vi "main.vi"() -> ()   [LabVIEW 2015]
uses:
  <vilib>/Bitlis-MEN/Parallel Stop/Software/Stop_Command.ctl
  test_chamber/Test Chamber/sub/MKS/Product/MFC/Type Definitions/Modbus Action.ctl
  <vilib>/Utility/file.llb/Write Delimited Spreadsheet (string).vi
  <vilib>/Utility/file.llb/Write Delimited Spreadsheet (DBL).vi
panel:
  in  "?":enum32{"Main", "Notes"}(tab)
  in  "submit_note":bool
  out "pv_6":dbl format="%#_3f"
  in  "sp_6":dbl
  in  "slide_6":dbl(slide) scale=0.0..500.0 scale format="%#_6p"
  out "label_6":string
  out "pv_5":dbl format="%#_3f"
  in  "sp_5":dbl
  in  "slide_5":dbl(slide) scale=0.0..500.0 scale format="%#_6p"
  out "label_5":string
  out "pv_4":dbl format="%#_3f"
  in  "sp_4":dbl
  in  "slide_4":dbl(slide) scale=0.0..500.0 scale format="%#_6p"
  out "label_4":string
  out "pv_3":dbl format="%#_3f"
  in  "sp_3":dbl
  in  "slide_3":dbl(slide) scale=0.0..500.0 scale format="%#_6p"
  out "label_3":string
  out "pv_2":dbl format="%#_3f"
  in  "sp_2":dbl
  in  "slide_2":dbl(slide) scale=0.0..10000.0 scale format="%#_1p"
  out "label_2":string
  out "pv_1":dbl format="%#_3f"
  in  "sp_1":dbl
  in  "slide_1":dbl(slide) scale=0.0..20000.0 scale format="%#_6p"
  out "label_1":string
  in  "mfc_activated 6":bool
  in  "mfc_ip 6":string="192.168.2.6"
  in  "mfc_ip 5":string="192.168.2.5"
  in  "mfc_ip 4":string="192.168.2.4"
  in  "mfc_ip 3":string="192.168.2.3"
  in  "mfc_ip 2":string="192.168.2.2"
  in  "mfc_ip1":string="192.168.2.1"
  in  "mfc_label 6":string="MFC6"
  in  "mfc_label 5":string="MFC5"
  in  "mfc_label 4":string="MFC4"
  in  "mfc_label 3":string="MFC3"
  in  "mfc_label 2":string="MFC 2"
  in  "mfc_label1":string="MFC 1"
  in  "mfc_activated 5":bool
  in  "mfc_activated 4":bool
  in  "mfc_activated 3":bool
  in  "mfc_activated 2":bool
  in  "mfc_activated1":bool
  out "?":errorcluster
  in  "Stop Button":bool
  out "Current State":T1(ring)
  in  "freq":u32=250
  in  "Add a note":string
  in  "File Path Control":path=path "E:/MFC Logger"
  out "Notes":string[][](table)
  # "Things to do:\n\n1) Logging\n2) Note taking\n3) Calibration Page/Worksheet"
  # "Label"
  # "IP Address"
  # "Activated?"
  # "MFC 1"
  # "MFC 2"
  # "MFC 3"
  # "MFC 4"
  # "MFC 5"
  # "MFC 6"
  # "Timestamp"
  # "Message"
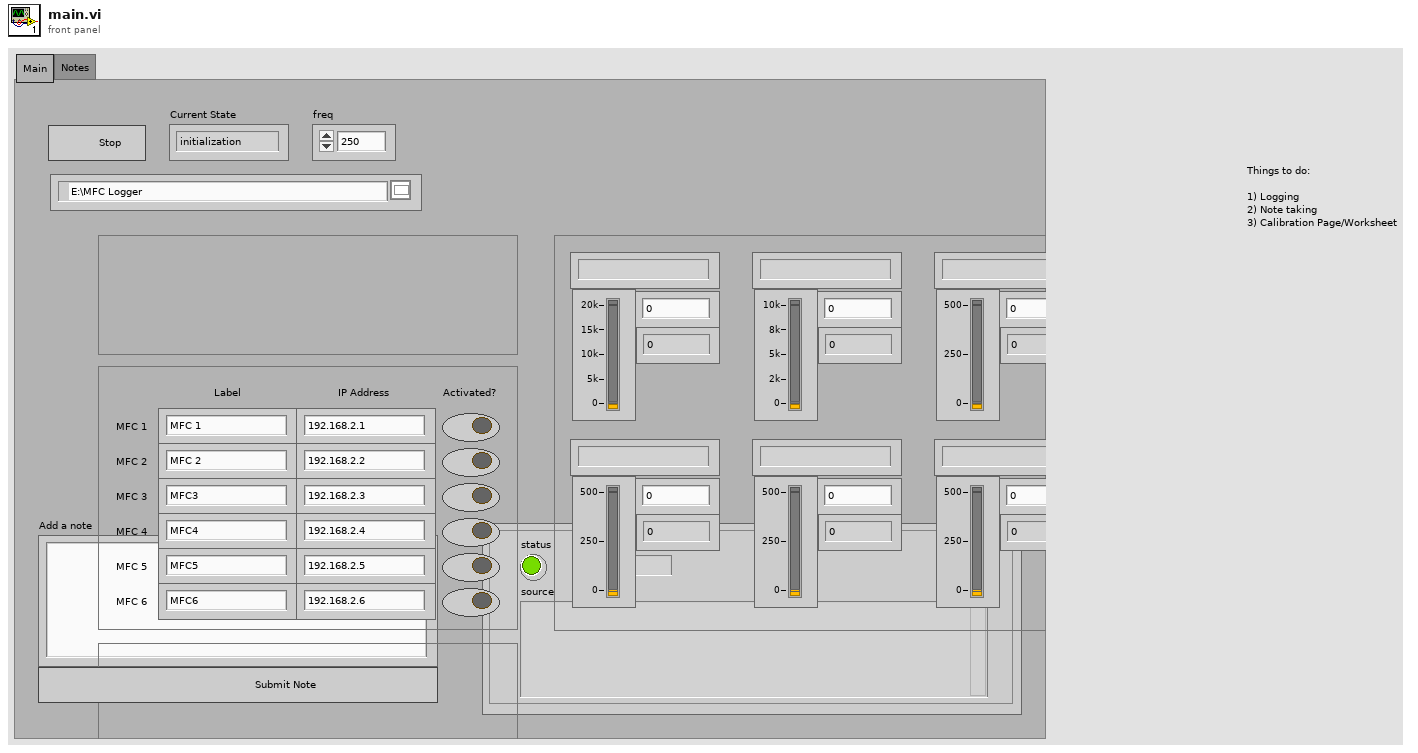
[diagram p1: front panel]
types:
  T1 = enum16{"initialization", "mode_selection", "auto_mode", "manual_mode", "safe_shutdown"}
  T2 = cluster{"Label":string, "IP":string, "Enabled":bool, "TCP Ref":refnum<k5>}[]
  T3 = cluster{"Label":string, "IP":string, "Enabled":bool, "TCP Ref":refnum<k5>}
  T4 = typedef "Stop_Command.ctl" = enum16{"Reset", "Read", "Write", "Close"}
  T5 = typedef "Modbus Action.ctl" = enum16{"Read", "Write"}
  T6 = enum8{"Enabled", "Disabled", "Disabled and Grayed Out"}
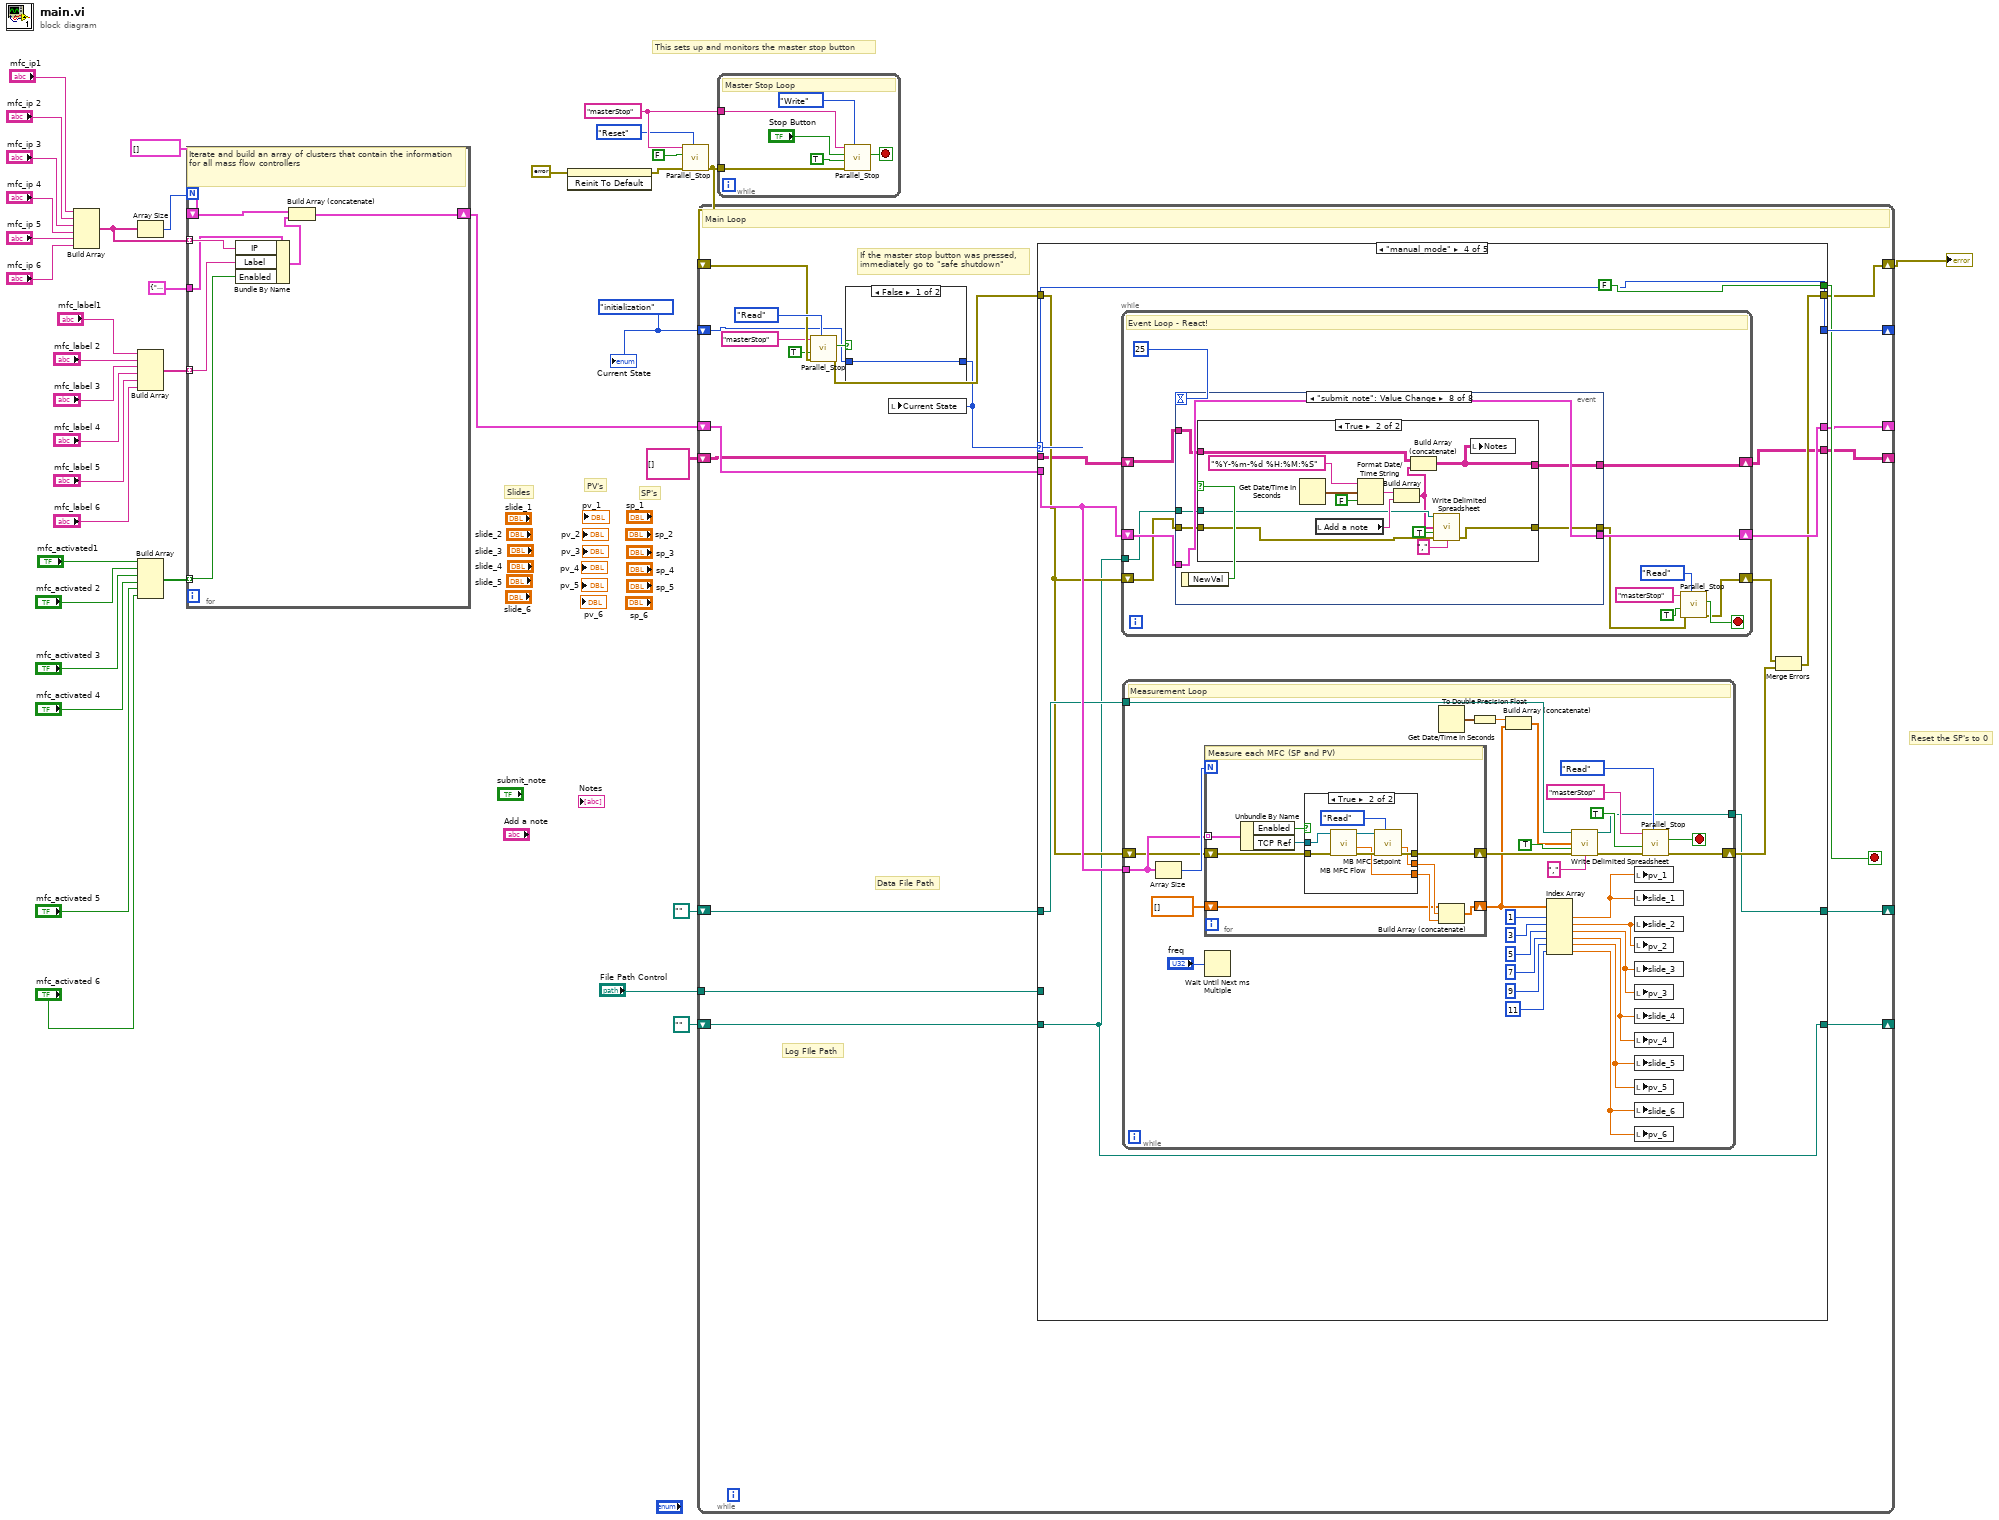
[diagram p0: block diagram]
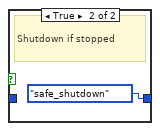
[diagram p2: hidden frame]
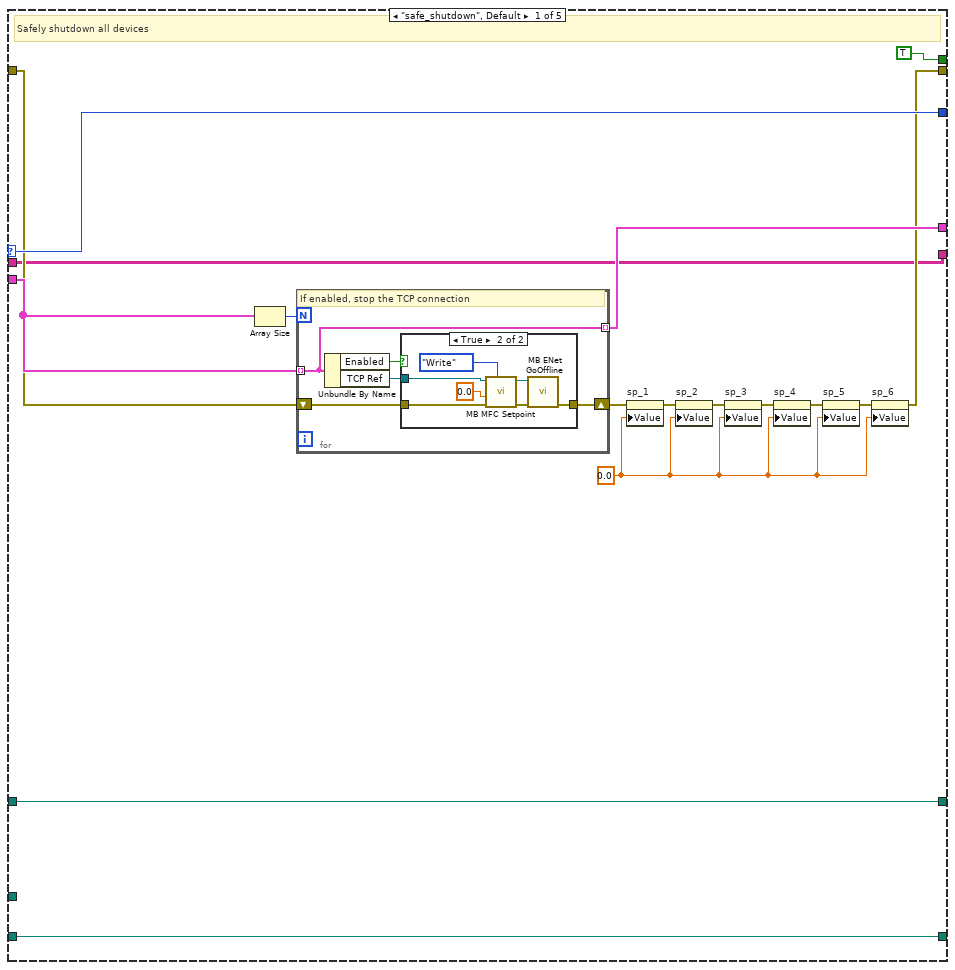
[diagram p3: hidden frame]
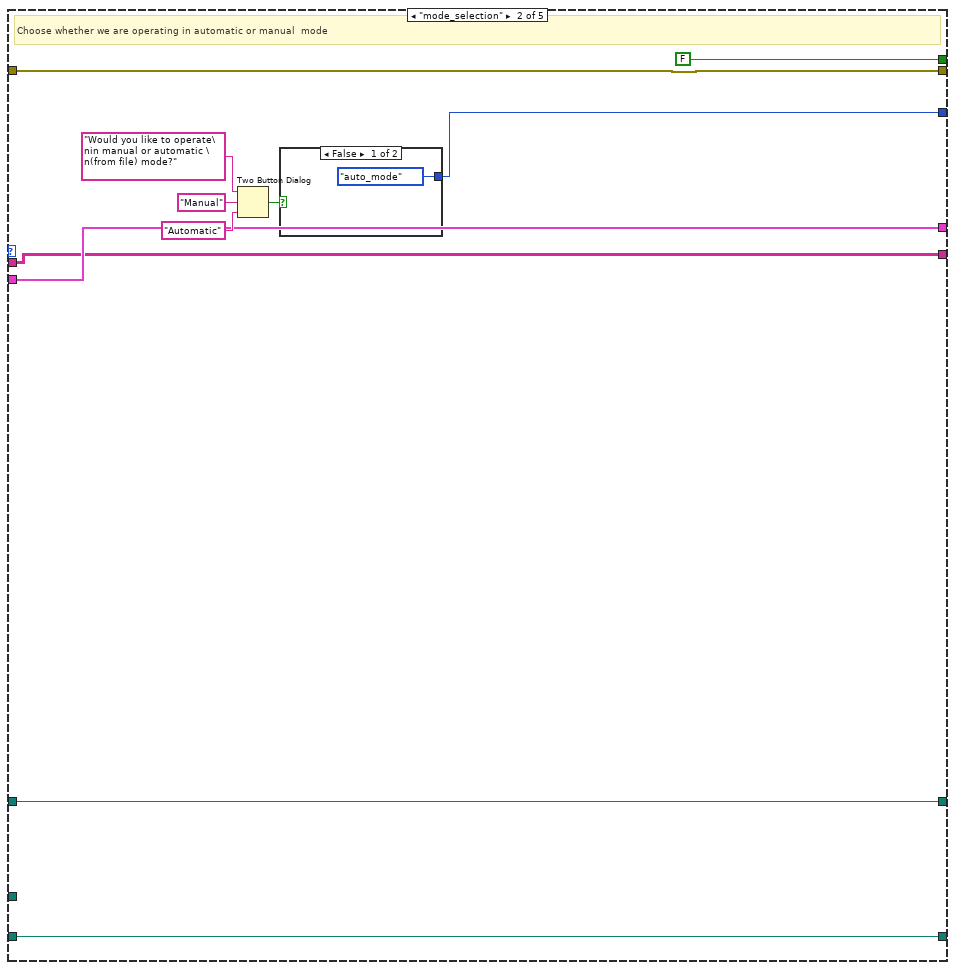
[diagram p5: hidden frame]
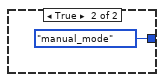
[diagram p6: hidden frame]
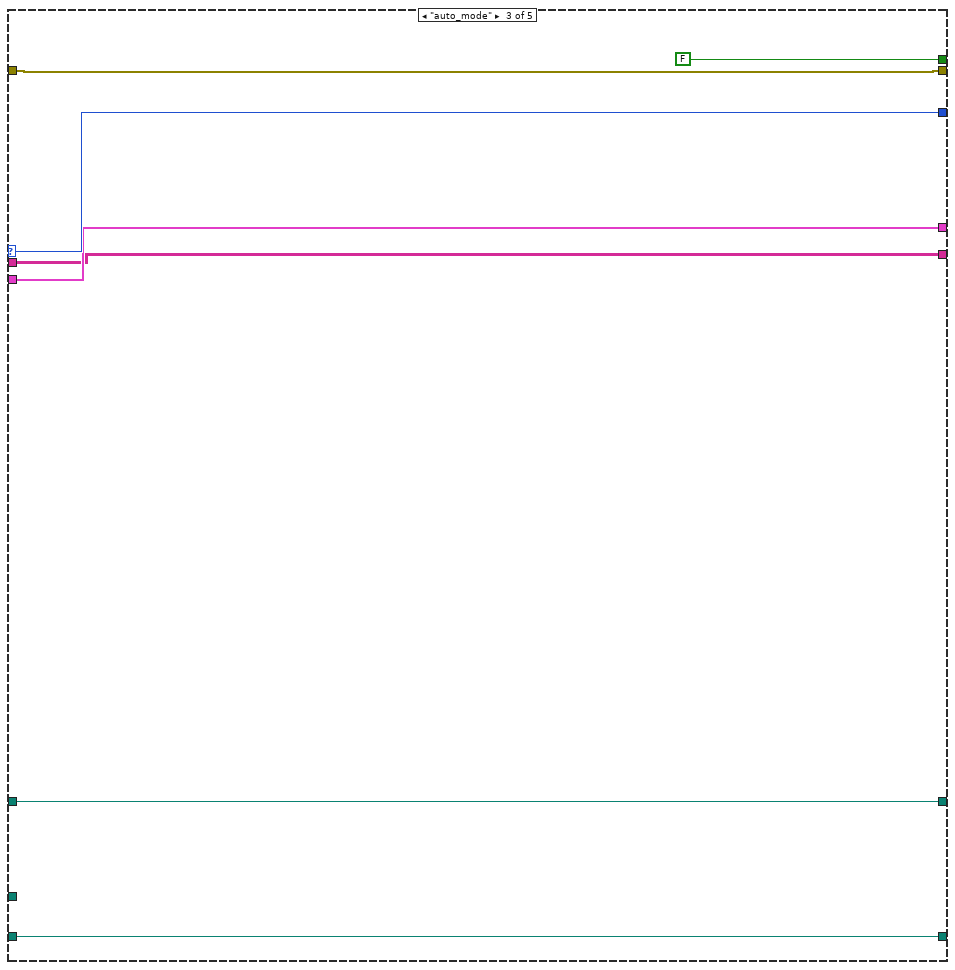
[diagram p7: hidden frame]
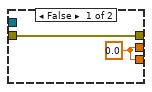
[diagram p8: hidden frame]
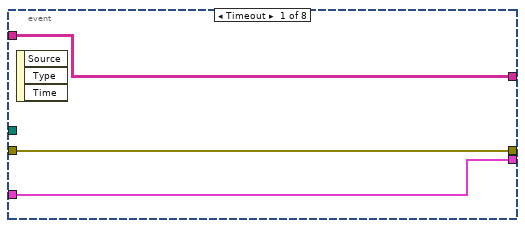
[diagram p9: hidden frame]
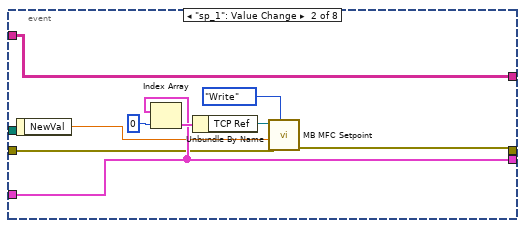
[diagram p10: hidden frame]
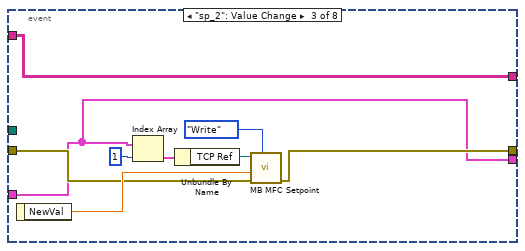
[diagram p11: hidden frame]
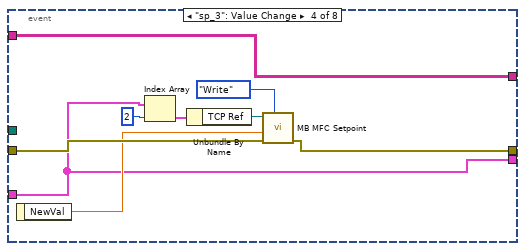
[diagram p12: hidden frame]
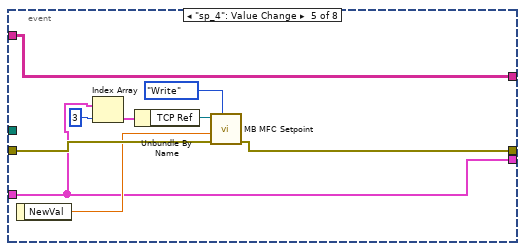
[diagram p13: hidden frame]
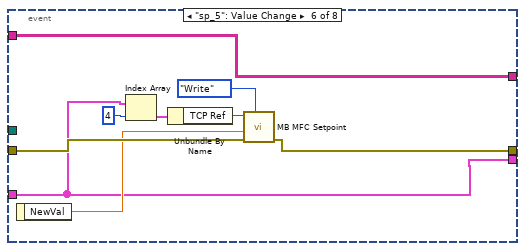
[diagram p14: hidden frame]
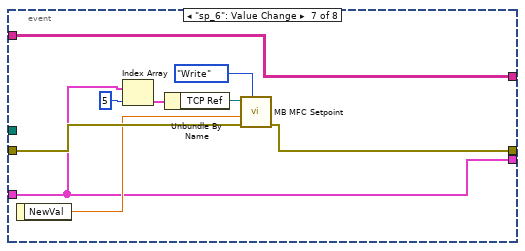
[diagram p15: hidden frame]
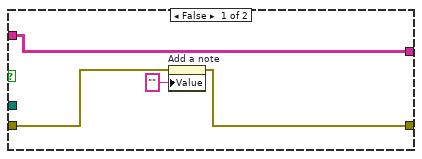
[diagram p16: hidden frame]
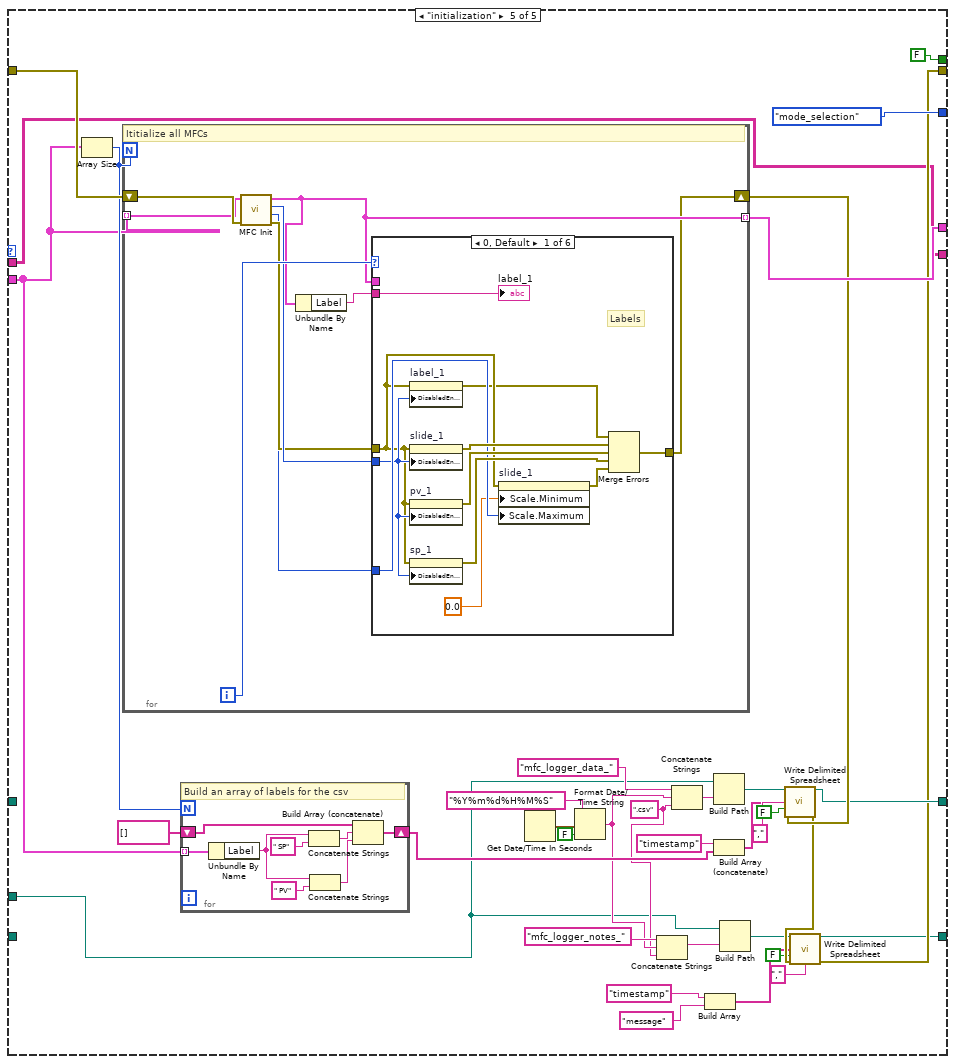
[diagram p17: hidden frame]
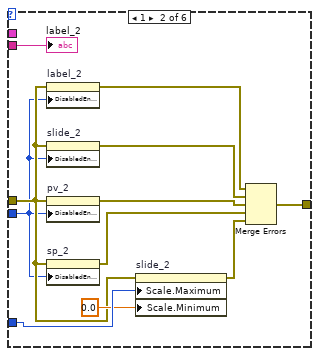
[diagram p18: hidden frame]
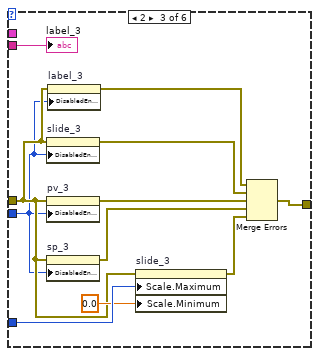
[diagram p19: hidden frame]
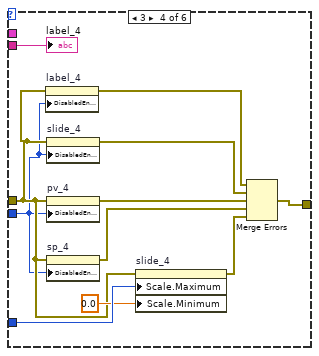
[diagram p20: hidden frame]
diagram:
  w37 = "masterStop" ("Name")
  w31 = T1."initialization"
  # "Reset the SP's to 0"
  # "SP's"
  # "PV's"
  # "Slides"
  # "This sets up and monitors the master stop button"
  n1 = Build Array("mfc_ip1", "mfc_ip 2", "mfc_ip 3", "mfc_ip 4", "mfc_ip 5", "mfc_ip 6") -> (w10:string[])
  n2 = Array Size(array=w10) -> (size(s)=w11:i32)
  n3 = Build Array("mfc_label1", "mfc_label 2", "mfc_label 3", "mfc_label 4", "mfc_label 5", "mfc_label 6") -> (w9:string[])
  n4 = Build Array("mfc_activated1", "mfc_activated 2", "mfc_activated 3", "mfc_activated 4", "mfc_activated 5", "mfc_activated 6") -> (w8:bool[])
  n5 = for {
    N: w11 -> [_]
    tunnel: w10 -> [w44] mode=indexing
    tunnel: w9 -> [w43] mode=indexing
    tunnel: w8 -> [w42] mode=indexing
    shift-right: [w41] -> w7
    shift-left: T2 [] -> [w39]
    tunnel: T3 {"Label"="192.168.2.6", "IP"="MFC6", "Enabled"=FALSE, "TCP Ref"=refnum} ("Cluster in") -> [w38]
    # "Iterate and build an array of clusters that contain the information for all mass flow controllers"
    n6 = Bundle By Name(cluster=w38, "IP"=w44, "Label"=w43, "Enabled"=w42) -> (w40:T3)
    n7 = Build Array (concatenate)(w39, w40) -> (w41:T2)
  }
  n8 = invoke class="Clust (strict)" method="Reinit To Default"(error in=errorcluster {"status"=FALSE, "code"=0, "source"=""} ("error in (no error)")) -> (error out=w32:errorcluster)  [unwired: 2 in, 2 out]
  n9 = call <vilib>:"Parallel_Stop.vi"("Command"=Stop_Command."Reset", "error in (no error)"=w32, "Stop?"=FALSE, "Name"=w37) -> ("error out"=w30:errorcluster)  [unwired: 6 in, 1 out]
  n10 = while {
    shift-right: [w54] -> w34
    shift-left: w30 -> [w63]
    shift-right: [w57] -> _
    shift-left: w31 -> [w59]
    shift-right: [w52] -> _
    shift-left: w7 -> [w53]
    tunnel: "File Path Control" -> [w51]
    shift-right: [w50] -> _
    shift-left: path "" ("new file path (Not A Path if cancelled)") -> [w49]
    shift-right: [w47] -> _
    shift-left: path "" ("new file path (Not A Path if cancelled)") -> [w48]
    shift-right: [w46] -> _
    shift-left: string[][] [] -> [w45]
    stop <- w55 stop-if-true
    # "Data File Path"
    # "Log FIle Path"
    # "If the master stop button was pressed,\nimmediately go to \"safe shutdown\""
    # "Main Loop"
    n11 = call <vilib>:"Parallel_Stop.vi"("Command"=Stop_Command."Read", "error in (no error)"=w63, "Stop on Error? (T)"=TRUE, "Name"="masterStop") -> ("error out"=w62:errorcluster, "Latched Stop"=w60:bool)  [unwired: 6 in]
    n12 = case shown="False" w60 {
      tunnel: [w65 T1."safe_shutdown"] -> w56
      tunnel: w59 -> [w65 _]
      frame False {
      }
      frame True {
        # "Shutdown if stopped"
      }
    }
    n13 = local write "Current State"(w56) -> ()
    n14 = case shown="\"manual_mode\"" w56 {
      selector: w56 -> [w83 _ w116 w128 _]
      tunnel: w62 -> [w78 w107 w115 w120 w306]
      tunnel: [w70 w107 w115 w125 w288] -> w54
      tunnel: [w83 w101 w116 w128 T1."mode_selection"] -> w57
      tunnel: [TRUE FALSE FALSE FALSE FALSE] -> w55
      tunnel: [w79 w100 w113 w127 w307] -> w52
      tunnel: w53 -> [w80 w100 w113 w123 w295]
      tunnel: w51 -> [_ _ _ _ w278]
      tunnel: [w69 w99 w112 w121 w299] -> w50
      tunnel: w49 -> [w69 w99 w112 w122 _]
      tunnel: w48 -> [w68 w98 w111 w119 _]
      tunnel: [w68 w98 w111 w119 w277] -> w47
      tunnel: [w67 w97 w110 w118 w275] -> w46
      tunnel: w45 -> [w67 w97 w110 w117 w275]
      frame "safe_shutdown", Default {
        w71 = 0.0 ("sp_1")
        # "Safely shutdown all devices"
        n15 = Array Size(array=w80) -> (size(s)=w81:i32)
        n16 = for {
          N: w81 -> [_]
          tunnel: w80 -> [w87] mode=indexing
          tunnel: [w87] -> w79 mode=indexing
          shift-right: [w85] -> w77
          shift-left: w78 -> [w86]
          # "If enabled, stop the TCP connection"
          n17 = Unbundle By Name(w87) -> ("Enabled"=w88:bool, "TCP Ref"=w84:refnum<k5>)
          n18 = case shown="True" w88 {
            tunnel: w86 -> [w89 w96]
            tunnel: [w89 w91] -> w85
            tunnel: w84 -> [_ w94]
            frame False {
            }
            frame True {
              n19 = call "MB MFC Setpoint.vi"("Action"=Modbus_Action."Write", "error in (no error)"=w96, "Setpoint"=sgl 0.0, "TCP Ref"=w94) -> ("error out"=w92:errorcluster, "dup TCP Ref"=w90:refnum<k5>)  [unwired: 5 in, 1 out]
              n20 = call "MB ENet GoOffline.vi"("error in (no error)"=w92, "TCP Ref:ValBlock"=w90) -> ("error out"=w91:errorcluster)  [unwired: 7 in, 2 out]
            }
          }
        }
        n21 = property on="sp_1" class="DigNum (strict)"(error in=w77, "Value"=w71) -> (error out=w76:errorcluster)  [unwired: 1 in, 1 out]
        n22 = property on="sp_2" class="DigNum (strict)"(error in=w76, "Value"=w71) -> (error out=w75:errorcluster)  [unwired: 1 in, 1 out]
        n23 = property on="sp_3" class="DigNum (strict)"(error in=w75, "Value"=w71) -> (error out=w74:errorcluster)  [unwired: 1 in, 1 out]
        n24 = property on="sp_4" class="DigNum (strict)"(error in=w74, "Value"=w71) -> (error out=w73:errorcluster)  [unwired: 1 in, 1 out]
        n25 = property on="sp_5" class="DigNum (strict)"(error in=w73, "Value"=w71) -> (error out=w72:errorcluster)  [unwired: 1 in, 1 out]
        n26 = property on="sp_6" class="DigNum (strict)"(error in=w72, "Value"=w71) -> (error out=w70:errorcluster)  [unwired: 1 in, 1 out]
      }
      frame "mode_selection" {
        # "Choose whether we are operating in automatic or manual  mode"
        n27 = Two Button Dialog(message="Would you like to operate\nin manual or automatic \n(from file) mode?", 1:"Automatic" ("F button name (\"Cancel\")"), 2:"Manual" ("T button name (\"OK\")")) -> (T button?=w102:bool)
        n28 = case shown="False" w102 {
          tunnel: [T1."auto_mode" T1."manual_mode"] -> w101
          frame False {
          }
          frame True {
          }
        }
      }
      frame "auto_mode" {
      }
      frame "manual_mode" {
        n29 = while {
          shift-right: [w186] -> w127
          shift-left: w123 -> [w187]
          shift-right: [w189] -> w126
          shift-left: w120 -> [w184]
          tunnel: w119 -> [w183]
          shift-right: [w182] -> w118
          shift-left: w117 -> [w181]
          stop <- w193 stop-if-true
          # "Event Loop - React!"
          n30 = event shown="[7] \"submit_note\": Value Change" {
            selector: _ -> [_ _ _ _ _ _ _ _]
            dyn-events: _ -> [_ _ _ _ _ _ _ _]
            timeout: 25 -> [_ _ _ _ _ _ _ _]
            tunnel: w187 -> [w195 w201 w207 w216 w228 w237 w246 w256]
            tunnel: [w195 w201 w207 w216 w228 w237 w246 w256] -> w186
            tunnel: w184 -> [w196 w200 w213 w222 w231 w241 w249 w255]
            tunnel: [w196 w199 w212 w223 w232 w240 w250 w254] -> w185
            tunnel: w183 -> [_ _ _ _ _ _ _ w253]
            tunnel: [w194 w197 w206 w215 w224 w233 w242 w252] -> w182
            tunnel: w181 -> [w194 w197 w206 w215 w224 w233 w242 w251]
            event Timeout {
              n31 = event-data() -> ()  [unwired: 1 in, 3 out]
            }
            event "sp_1": Value Change {
              n32 = event-data() -> ("NewVal"=w198:dbl)  [unwired: 1 in]
              n33 = Index Array(array=w201, index=0) -> (element=w203:T3)
              n34 = Unbundle By Name(w203) -> ("TCP Ref"=w202:refnum<k5>)
              n35 = call "MB MFC Setpoint.vi"("Action"=Modbus_Action."Write", "error in (no error)"=w200, "Setpoint"=w198, "TCP Ref"=w202) -> ("error out"=w199:errorcluster)  [unwired: 5 in, 2 out]
            }
            event "sp_2": Value Change {
              n36 = event-data() -> ("NewVal"=w214:dbl)  [unwired: 1 in]
              n37 = Index Array(array=w207, index=1) -> (element=w210:T3)
              n38 = Unbundle By Name(w210) -> ("TCP Ref"=w209:refnum<k5>)
              n39 = call "MB MFC Setpoint.vi"("Action"=Modbus_Action."Write", "error in (no error)"=w213, "Setpoint"=w214, "TCP Ref"=w209) -> ("error out"=w212:errorcluster)  [unwired: 5 in, 2 out]
            }
            event "sp_3": Value Change {
              n40 = event-data() -> ("NewVal"=w221:dbl)  [unwired: 1 in]
              n41 = Index Array(array=w216, index=2) -> (element=w218:T3)
              n42 = Unbundle By Name(w218) -> ("TCP Ref"=w217:refnum<k5>)
              n43 = call "MB MFC Setpoint.vi"("Action"=Modbus_Action."Write", "error in (no error)"=w222, "Setpoint"=w221, "TCP Ref"=w217) -> ("error out"=w223:errorcluster)  [unwired: 5 in, 2 out]
            }
            event "sp_4": Value Change {
              n44 = event-data() -> ("NewVal"=w230:dbl)  [unwired: 1 in]
              n45 = Index Array(array=w228, index=3) -> (element=w226:T3)
              n46 = Unbundle By Name(w226) -> ("TCP Ref"=w225:refnum<k5>)
              n47 = call "MB MFC Setpoint.vi"("Action"=Modbus_Action."Write", "error in (no error)"=w231, "Setpoint"=w230, "TCP Ref"=w225) -> ("error out"=w232:errorcluster)  [unwired: 5 in, 2 out]
            }
            event "sp_5": Value Change {
              n48 = event-data() -> ("NewVal"=w239:dbl)  [unwired: 1 in]
              n49 = Index Array(array=w237, index=4) -> (element=w235:T3)
              n50 = Unbundle By Name(w235) -> ("TCP Ref"=w234:refnum<k5>)
              n51 = call "MB MFC Setpoint.vi"("Action"=Modbus_Action."Write", "error in (no error)"=w241, "Setpoint"=w239, "TCP Ref"=w234) -> ("error out"=w240:errorcluster)  [unwired: 5 in, 2 out]
            }
            event "sp_6": Value Change {
              n52 = event-data() -> ("NewVal"=w248:dbl)  [unwired: 1 in]
              n53 = Index Array(array=w246, index=5) -> (element=w244:T3)
              n54 = Unbundle By Name(w244) -> ("TCP Ref"=w243:refnum<k5>)
              n55 = call "MB MFC Setpoint.vi"("Action"=Modbus_Action."Write", "error in (no error)"=w249, "Setpoint"=w248, "TCP Ref"=w243) -> ("error out"=w250:errorcluster)  [unwired: 5 in, 2 out]
            }
            event "submit_note": Value Change {
              n56 = event-data() -> ("NewVal"=w257:bool)  [unwired: 1 in]
              n57 = case shown="True" w257 {
                tunnel: w255 -> [w260 w269]
                tunnel: [w259 w268] -> w254
                tunnel: w253 -> [_ w265]
                tunnel: [w258 w262] -> w252
                tunnel: w251 -> [w258 w264]
                frame False {
                  n58 = property on="Add a note" class="Str"(error in=w260, "Value"="" ("Add a note")) -> (error out=w259:errorcluster)  [unwired: 1 in, 1 out]
                }
                frame True {
                  n59 = Get Date/Time In Seconds() -> (seconds since 1Jan1904=w271:timestamp)
                  n60 = local read "Add a note"() -> (w270:string)
                  n61 = Format Date/Time String(time format string (%c)="%Y-%m-%d %H:%M:%S", seconds (now)=w271, UTC format=FALSE) -> (date/time string=w274:string)
                  n62 = Build Array(w274, w270) -> (w263:string[])
                  n63 = Build Array (concatenate)(w264, w263) -> (w262:string[][])
                  n64 = call-poly <vilib>:"Write Delimited Spreadsheet.vi"("file path (dialog if empty)"=w265, "1D data"=w263, "append to file? (F)"=TRUE, "error in (no error)"=w269, "delimiter (\\t)"="," ("delimiter (\\t)")) -> ("error out"=w268:errorcluster)  [unwired: 9 in, 1 out]
                  n65 = local write "Notes"(w262) -> ()
                }
              }
            }
          }
          n66 = call <vilib>:"Parallel_Stop.vi"("Command"=Stop_Command."Read", "error in (no error)"=w185, "Stop on Error? (T)"=TRUE, "Name"="masterStop") -> ("error out"=w189:errorcluster, "Latched Stop"=w193:bool)  [unwired: 6 in]
        }
        n67 = while {
          shift-right: [w160] -> w124
          shift-left: w120 -> [w154]
          tunnel: w123 -> [w155]
          tunnel: w122 -> [w135]
          tunnel: [w134] -> w121
          stop <- w161 stop-if-true
          # "Measurement Loop"
          n68 = Array Size(array=w155) -> (size(s)=w156:i32)
          n69 = for {
            N: w156 -> [_]
            tunnel: w155 -> [w170] mode=indexing
            shift-right: [w167] -> w139
            shift-left: w154 -> [w168]
            shift-right: [w163] -> w133
            shift-left: sgl[] [] -> [w162]
            # "Measure each MFC (SP and PV)"
            n70 = Unbundle By Name(w170) -> ("Enabled"=w169:bool, "TCP Ref"=w166:refnum<k5>)
            n71 = case shown="True" w169 {
              tunnel: w168 -> [w172 w180]
              tunnel: [w172 w177] -> w167
              tunnel: w166 -> [_ w179]
              tunnel: [w171 w174] -> w165
              tunnel: [w171 w173] -> w164
              frame False {
                w171 = 0.0 ("element")
              }
              frame True {
                n72 = call "MB MFC Flow.vi"("error in (no error)"=w180, "TCP Ref"=w179) -> ("error out"=w178:errorcluster, "Flow(sccm)"=w174:sgl, "dup TCP Ref"=w176:refnum<k5>)  [unwired: 7 in]
                n73 = call "MB MFC Setpoint.vi"("Action"=Modbus_Action."Read", "error in (no error)"=w178, "TCP Ref"=w176) -> ("error out"=w177:errorcluster, "Setpoint"=w173:sgl)  [unwired: 6 in, 1 out]
              }
            }
            n74 = Build Array (concatenate)(w162, w164, w165) -> (w163:dbl[])
          }
          n75 = Wait Until Next ms Multiple(millisecond multiple="freq") -> ()  [unwired: 1 out]
          n76 = Get Date/Time In Seconds() -> (seconds since 1Jan1904=w131:timestamp)
          n77 = To Double Precision Float(number=w131) -> (double precision float=w132:dbl)
          n78 = Build Array (concatenate)(w132, w133) -> (w130:dbl[])
          n79 = Index Array(array=w133, index #1=1 ("index"), index #2=3 ("index"), index #3=5 ("index"), index #4=7 ("index"), index #5=9 ("index"), index #6=11 ("index")) -> (element #1=w147:dbl, element #2=w145:dbl, element #3=w144:dbl, element #4=w143:dbl, element #5=w142:dbl, element #6=w141:dbl)
          n80 = call-poly <vilib>:"Write Delimited Spreadsheet.vi"("file path (dialog if empty)"=w135, "1D data"=w130, "append to file? (F)"=TRUE, "error in (no error)"=w139, "delimiter (\\t)"="," ("delimiter (\\t)")) -> ("new file path (Not A Path if cancelled)"=w134:path, "error out"=w138:errorcluster)  [unwired: 9 in]
          n81 = local write "pv_1"(w147) -> ()
          n82 = local write "slide_1"(w147) -> ()
          n83 = local write "slide_2"(w145) -> ()
          n84 = local write "pv_2"(w145) -> ()
          n85 = local write "slide_3"(w144) -> ()
          n86 = local write "pv_3"(w144) -> ()
          n87 = local write "slide_4"(w143) -> ()
          n88 = local write "pv_4"(w143) -> ()
          n89 = local write "slide_5"(w142) -> ()
          n90 = local write "pv_5"(w142) -> ()
          n91 = local write "slide_6"(w141) -> ()
          n92 = local write "pv_6"(w141) -> ()
          n93 = call <vilib>:"Parallel_Stop.vi"("Command"=Stop_Command."Read", "error in (no error)"=w138, "Stop on Error? (T)"=TRUE, "Name"="masterStop") -> ("error out"=w160:errorcluster, "Latched Stop"=w161:bool)  [unwired: 6 in]
        }
        n94 = Merge Errors(w126, w124) -> (w125:errorcluster)
      }
      frame "initialization" {
        w284 = ".csv" ("string")
        n95 = Array Size(array=w295) -> (size(s)=w296:i32)
        n96 = for {
          N: w296 -> [_]
          tunnel: [w325] -> w307 mode=indexing
          shift-right: [w320] -> w305
          shift-left: w306 -> [w322]
          tunnel: w295 -> [w318] mode=indexing
          i -> [w326]
          # "Ititialize all MFCs"
          n97 = call "MFC Init.vi"("error in (no error)"=w322, "Cluster in"=w318) -> ("error out"=w321:errorcluster, "MFC Range"=w319:i32, "Disabled"=w323:T6, "Cluster out"=w325:T3)  [unwired: 6 in]
          n98 = Unbundle By Name(w325) -> ("Label"=w324:string)
          n99 = case shown="0, Default" w326 {
            tunnel: w325 -> [_ _ _ _ _ _]
            tunnel: w324 -> [w337 w348 w359 w370 w381 w392]
            tunnel: w323 -> [w329 w339 w349 w361 w371 w382]
            tunnel: w321 -> [w328 w340 w350 w362 w374 w384]
            tunnel: [w335 w347 w358 w369 w380 w391] -> w320
            tunnel: w319 -> [w331 w343 w354 w366 w376 w386]
            frame 0, Default {
              # "Labels"
              n100 = property on="label_1" class="Str"(error in=w328, "DisabledEnum"=w329) -> (error out=w327:errorcluster)  [unwired: 1 in, 1 out]
              n101 = property on="slide_1" class="Slide (strict)"(error in=w328, "DisabledEnum"=w329) -> (error out=w336:errorcluster)  [unwired: 1 in, 1 out]
              n102 = property on="pv_1" class="DigNum (strict)"(error in=w328, "DisabledEnum"=w329) -> (error out=w334:errorcluster)  [unwired: 1 in, 1 out]
              n103 = property on="sp_1" class="DigNum (strict)"(error in=w328, "DisabledEnum"=w329) -> (error out=w333:errorcluster)  [unwired: 1 in, 1 out]
              n104 = property on="slide_1" class="Slide (strict)"(error in=w328, "Scale.Minimum"=0.0 ("Scale.Range:Minimum"), "Scale.Maximum"=w331) -> (error out=w332:errorcluster)  [unwired: 1 in, 1 out]
              n105 = Merge Errors(w327, w336, w334, w333, w332) -> (w335:errorcluster)
              "label_1" <- w337
            }
            frame 1 {
              n106 = property on="label_2" class="Str"(error in=w340, "DisabledEnum"=w339) -> (error out=w338:errorcluster)  [unwired: 1 in, 1 out]
              n107 = property on="slide_2" class="Slide (strict)"(error in=w340, "DisabledEnum"=w339) -> (error out=w346:errorcluster)  [unwired: 1 in, 1 out]
              n108 = property on="pv_2" class="DigNum (strict)"(error in=w340, "DisabledEnum"=w339) -> (error out=w345:errorcluster)  [unwired: 1 in, 1 out]
              n109 = property on="sp_2" class="DigNum (strict)"(error in=w340, "DisabledEnum"=w339) -> (error out=w344:errorcluster)  [unwired: 1 in, 1 out]
              n110 = property on="slide_2" class="Slide (strict)"(error in=w340, "Scale.Maximum"=w343, "Scale.Minimum"=0.0 ("Scale.Range:Minimum")) -> (error out=w342:errorcluster)  [unwired: 1 in, 1 out]
              n111 = Merge Errors(w338, w346, w345, w344, w342) -> (w347:errorcluster)
              "label_2" <- w348
            }
            frame 2 {
              n112 = property on="slide_3" class="Slide (strict)"(error in=w350, "DisabledEnum"=w349) -> (error out=w357:errorcluster)  [unwired: 1 in, 1 out]
              n113 = property on="pv_3" class="DigNum (strict)"(error in=w350, "DisabledEnum"=w349) -> (error out=w356:errorcluster)  [unwired: 1 in, 1 out]
              n114 = property on="sp_3" class="DigNum (strict)"(error in=w350, "DisabledEnum"=w349) -> (error out=w355:errorcluster)  [unwired: 1 in, 1 out]
              n115 = property on="label_3" class="Str"(error in=w350, "DisabledEnum"=w349) -> (error out=w351:errorcluster)  [unwired: 1 in, 1 out]
              n116 = property on="slide_3" class="Slide (strict)"(error in=w350, "Scale.Maximum"=w354, "Scale.Minimum"=0.0 ("Scale.Range:Minimum")) -> (error out=w353:errorcluster)  [unwired: 1 in, 1 out]
              n117 = Merge Errors(w351, w357, w356, w355, w353) -> (w358:errorcluster)
              "label_3" <- w359
            }
            frame 3 {
              n118 = property on="label_4" class="Str"(error in=w362, "DisabledEnum"=w361) -> (error out=w360:errorcluster)  [unwired: 1 in, 1 out]
              n119 = property on="slide_4" class="Slide (strict)"(error in=w362, "DisabledEnum"=w361) -> (error out=w367:errorcluster)  [unwired: 1 in, 1 out]
              n120 = property on="pv_4" class="DigNum (strict)"(error in=w362, "DisabledEnum"=w361) -> (error out=w364:errorcluster)  [unwired: 1 in, 1 out]
              n121 = property on="sp_4" class="DigNum (strict)"(error in=w362, "DisabledEnum"=w361) -> (error out=w363:errorcluster)  [unwired: 1 in, 1 out]
              n122 = property on="slide_4" class="Slide (strict)"(error in=w362, "Scale.Maximum"=w366, "Scale.Minimum"=0.0 ("Scale.Range:Minimum")) -> (error out=w368:errorcluster)  [unwired: 1 in, 1 out]
              n123 = Merge Errors(w360, w367, w364, w363, w368) -> (w369:errorcluster)
              "label_4" <- w370
            }
            frame 4 {
              n124 = property on="label_5" class="Str"(error in=w374, "DisabledEnum"=w371) -> (error out=w372:errorcluster)  [unwired: 1 in, 1 out]
              n125 = property on="slide_5" class="Slide (strict)"(error in=w374, "DisabledEnum"=w371) -> (error out=w373:errorcluster)  [unwired: 1 in, 1 out]
              n126 = property on="pv_5" class="DigNum (strict)"(error in=w374, "DisabledEnum"=w371) -> (error out=w379:errorcluster)  [unwired: 1 in, 1 out]
              n127 = property on="sp_5" class="DigNum (strict)"(error in=w374, "DisabledEnum"=w371) -> (error out=w378:errorcluster)  [unwired: 1 in, 1 out]
              n128 = property on="slide_5" class="Slide (strict)"(error in=w374, "Scale.Maximum"=w376, "Scale.Minimum"=0.0 ("Scale.Range:Minimum")) -> (error out=w377:errorcluster)  [unwired: 1 in, 1 out]
              n129 = Merge Errors(w372, w373, w379, w378, w377) -> (w380:errorcluster)
              "label_5" <- w381
            }
            frame 5 {
              n130 = property on="label_6" class="Str"(error in=w384, "DisabledEnum"=w382) -> (error out=w383:errorcluster)  [unwired: 1 in, 1 out]
              n131 = property on="slide_6" class="Slide (strict)"(error in=w384, "DisabledEnum"=w382) -> (error out=w390:errorcluster)  [unwired: 1 in, 1 out]
              n132 = property on="pv_6" class="DigNum (strict)"(error in=w384, "DisabledEnum"=w382) -> (error out=w389:errorcluster)  [unwired: 1 in, 1 out]
              n133 = property on="sp_6" class="DigNum (strict)"(error in=w384, "DisabledEnum"=w382) -> (error out=w388:errorcluster)  [unwired: 1 in, 1 out]
              n134 = property on="slide_6" class="Slide (strict)"(error in=w384, "Scale.Maximum"=w386, "Scale.Minimum"=0.0 ("Scale.Range:Minimum")) -> (error out=w387:errorcluster)  [unwired: 1 in, 1 out]
              n135 = Merge Errors(w383, w390, w389, w388, w387) -> (w391:errorcluster)
              "label_6" <- w392
            }
          }
        }
        n136 = for {
          N: w296 -> [_]
          tunnel: w295 -> [w317] mode=indexing
          shift-right: [w311] -> w293
          shift-left: string[] [] -> [w310]
          # "Build an array of labels for the csv"
          n137 = Unbundle By Name(w317) -> ("Label"=w316:string)
          n138 = Concatenate Strings(w316, " SP" ("string")) -> (w313:string)
          n139 = Concatenate Strings(w316, " PV" ("string")) -> (w312:string)
          n140 = Build Array (concatenate)(w310, w313, w312) -> (w311:string[])
        }
        n141 = Get Date/Time In Seconds() -> (seconds since 1Jan1904=w292:timestamp)
        n142 = Format Date/Time String(time format string (%c)="%Y%m%d%H%M%S", seconds (now)=w292, UTC format=FALSE) -> (date/time string=w285:string)
        n143 = Concatenate Strings("mfc_logger_notes_" ("name or relative path"), w285, w284) -> (w283:string)
        n144 = Concatenate Strings("mfc_logger_data_" ("name or relative path"), w285, w284) -> (w301:string)
        n145 = Build Array("timestamp" ("name or relative path"), "message" ("name or relative path")) -> (w281:string[])
        n146 = Build Path(base path=w278, name or relative path=w301) -> (appended path=w300:path)
        n147 = Build Array (concatenate)("timestamp", w293) -> (w297:string[])
        n148 = Build Path(base path=w278, name or relative path=w283) -> (appended path=w282:path)
        n149 = call-poly <vilib>:"Write Delimited Spreadsheet.vi"("file path (dialog if empty)"=w300, "1D data"=w297, "append to file? (F)"=FALSE, "error in (no error)"=w305, "delimiter (\\t)"="," ("delimiter (\\t)")) -> ("new file path (Not A Path if cancelled)"=w299:path, "error out"=w289:errorcluster)  [unwired: 9 in]
        n150 = call-poly <vilib>:"Write Delimited Spreadsheet.vi"("file path (dialog if empty)"=w282, "1D data"=w281, "append to file? (F)"=FALSE, "error in (no error)"=w289, "delimiter (\\t)"="," ("delimiter (\\t)")) -> ("new file path (Not A Path if cancelled)"=w277:path, "error out"=w288:errorcluster)  [unwired: 9 in]
      }
    }
  }
  "?" <- w34
  n151 = while {
    tunnel: w30 -> [w398]
    tunnel: w37 -> [w393]
    stop <- w397 stop-if-true
    # "Master Stop Loop"
    n152 = call <vilib>:"Parallel_Stop.vi"("Command"=Stop_Command."Write", "error in (no error)"=w398, "Stop on Error? (T)"=TRUE, "Stop?"="Stop Button", "Name"=w393) -> ("Latched Stop"=w397:bool)  [unwired: 5 in, 1 out]
  }
  "Current State" <- w31
